vi "testSet.vi"(8 "error in (no error)":errorcluster) -> (0 "error out":errorcluster)   [LabVIEW 2019, in "AssertionTest.lvlib" / "AssertCount.lvlib"]
uses:
  AssertCount.lvlib
  Assertion/Assertion.lvlib
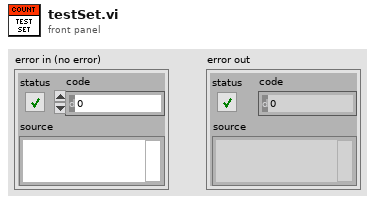
[diagram p1: front panel]
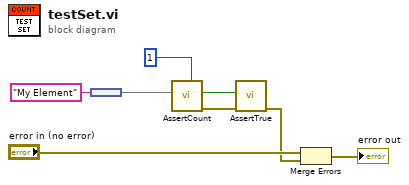
[diagram p0: block diagram]
diagram:
  n1 = node("My Element" ("element")) -> (w7:set{string})
  n2 = call "AssertCount.vi"("Expected"=1, "Haystack"=w7) -> ("error out"=w5:errorcluster, "Result"=w4:bool)  [unwired: 8 in]
  n3 = call "AssertTrue.vi"("error in (no error)"=w5, "Condition"=w4) -> ("error out"=w2:errorcluster)  [unwired: 8 in, 1 out]
  n4 = Merge Errors("error in (no error)", w2) -> (→"error out":errorcluster)
